vi "Stoerungen (449-512) - TRE08.vi"(8 "Fehler (Eingang)":errorcluster caption="Fehler (Eingang, kein Fehler)") -> (0 "Fehler (Ausgang)":errorcluster, 3 "Störungen 449-512":u64)   [LabVIEW 2015, in "Stoerungen.lvlib"]
uses:
  Stoerungen.lvlib
  PNS/Parameternamen PNS.ctl
  PNS/PNS.lvlib
  Stoerungen Messgeraet/Aktionen Kommunikation Stoerung.ctl
  Seiten/System Einstellungen/System Einstellungen.lvlib
  Seiten/System Einstellungen/Aktioen FGV System.ctl
  PNS/Aktionen FGV Istwerte.ctl
  cRIO/Stoermeldungen/Stoerungen 449-512.ctl
  cRIO/Stoermeldungen/Stoermeldungen.lvlib
panel:
  # "Störmeldungen PNS (449-512)"
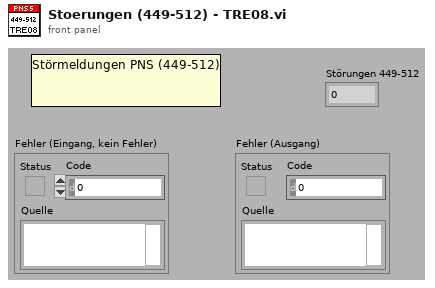
[diagram p1: front panel]
types:
  T1 = typedef "System Einstellungen.lvlib/Aktioen FGV System.ctl" = enum16{"lesen", "laden", "speichern", "Optionen schreiben", "Zeitstempel", "Reset BMP", "Reset SQP", "Wartung"}
  T2 = typedef "System Einstellungen.lvlib/Optionen.ctl" = cluster{"Störmeldep.":bool, "Betriebszustände":bool, "LN2 Befüllung":bool, "Klimaanlage ?":bool, "AK in ppm":bool, "log Cal-Gas":bool, "log 0-Gas":bool, "log CG zu PNS":bool, "Reserve":bool, "Reserve1":bool, "PNS?":bool, "Container":bool, "Mit N2 spülen":bool, "Span Gas Auswahl":T3, "VFS 1":bool, "VFS 2":bool, "VFS 3":bool, "VFS 4":bool, "TRE08":bool}
  T3 = typedef "Funktionstasten.lvlib/Spaneingang.ctl" = u16
  T4 = typedef "PNS.lvlib/Parameternamen PNS.ctl" = enum16{"Heizkreis 1", "Heizkreis 2", "Heizkreis 3", "Heizkreis 4", "Heizkreis 5", "Heizkreis 6", "Heizkreis 7", "Heizkreis 8"}
  T5 = typedef "PNS.lvlib/Aktionen FGV Istwerte.ctl" = enum16{"lesen", "initialisieren", "schreiben", "Störungen"}
  T6 = typedef "Stoerungen.lvlib/Aktionen Kommunikation Stoerung.ctl" = enum16{"lesen", "init", "FT-IR Komm", "FT-IR Betriebsart", "FT-IR Hintergrund", "cRIO Komm", "PNS Komm", "Dichtheitstest", "Life Bit", "FTIR Komm AK", "PMA Komm", "FID Komm", "PMA Cal", "FID Ch4 Cal", "FID THC Cal", "Cal Timeout", "VFS 1 Komm", "VFS 2 Komm", "VFS 3 Komm", "VFS 4 Komm", "TRE 08 Komm", "CG-Test vorzeitig", "CG-Test Span 1", "CG-Test Span 2", "CG-Test Span 3", "CG-Test Messgas", "CG-Test löschen", "Test", "Amium AK"}
  T7 = typedef "Stoermeldungen.lvlib/Stoerungen 449-512.ctl" = cluster{"ERR. 449":bool, "ERR. 450":bool, "ERR. 451":bool, "ERR. 452":bool, "ERR. 453":bool, "ERR. 454":bool, "ERR. 455":bool, "ERR. 456":bool, "ERR. 457":bool, "ERR. 458":bool, "ERR. 459":bool, "ERR. 460":bool, "ERR. 461":bool, "ERR. 462":bool, "ERR. 463":bool, "ERR. 464":bool, "ERR. 465":bool, "ERR. 466":bool, "ERR. 467":bool, "ERR. 468":bool, "ERR. 469":bool, "ERR. 470":bool, "ERR. 471":bool, "ERR. 472":bool, "ERR. 473":bool, "ERR. 474":bool, "ERR. 475":bool, "ERR. 476":bool, "ERR. 477":bool, "ERR. 478":bool, "ERR. 479":bool, "ERR. 480":bool, "ERR. 481":bool, "ERR. 482":bool, "ERR. 483":bool, "ERR. 484":bool, "ERR. 485":bool, "ERR. 486":bool, "ERR. 487":bool, "ERR. 488":bool, "ERR. 489":bool, "ERR. 490":bool, "ERR. 491":bool, "ERR. 492":bool, "ERR. 493":bool, "ERR. 494":bool, "ERR. 495":bool, "ERR. 496":bool, "ERR. 497":bool, "ERR. 498":bool, "ERR. 499":bool, "ERR. 500":bool, "ERR. 501":bool, "ERR. 502":bool, "ERR. 503":bool, "ERR. 504":bool, "ERR. 505":bool, "ERR. 506":bool, "ERR. 507":bool, "ERR. 508":bool, "ERR. 509":bool, "ERR. 510":bool, "ERR. 511":bool, "ERR. 512":bool}
  T8 = typedef "Steuerung PNS.lvclass/Regler.ctl" = cluster{"Istwert":i16, "Sollwert":i16, "Alarm MIN":i16, "Alarm MAX":i16, "Regler sperren":i16, "Analog Ausgang":i16}[]
  T9 = cluster{"Istwert":i16, "Sollwert":i16, "Alarm MIN":i16, "Alarm MAX":i16, "Regler sperren":i16, "Analog Ausgang":i16}
  T10 = typedef "Stoerungen.lvlib/Stoerungen Messgeraete.ctl" = cluster{"FT-IR Komm":bool, "FT-IR Betriebsart":bool, "FT-IR Hintergrundscan":bool, "Dichtheitstest":bool, "cRIO Komm":bool, "PNS Komm":bool, "Life Bit":bool, "FT-IR AK Komm":bool, "PMA Komm":bool, "FID Komm":bool, "PMA Cal":bool, "FID CH4 Cal":bool, "FID THC Cal":bool, "Cal Timeout":bool, "VFS 1 Komm":bool, "VFS 2 Komm":bool, "VFS 3 Komm":bool, "VFS 4 Komm":bool, "TRE 08 Komm":bool, "CG-Test":bool, "CG-Test 1":bool, "CG-Test 2":bool, "CG-Test 3":bool, "Messgas - Eingang":bool, "Amium AK Komm":bool}
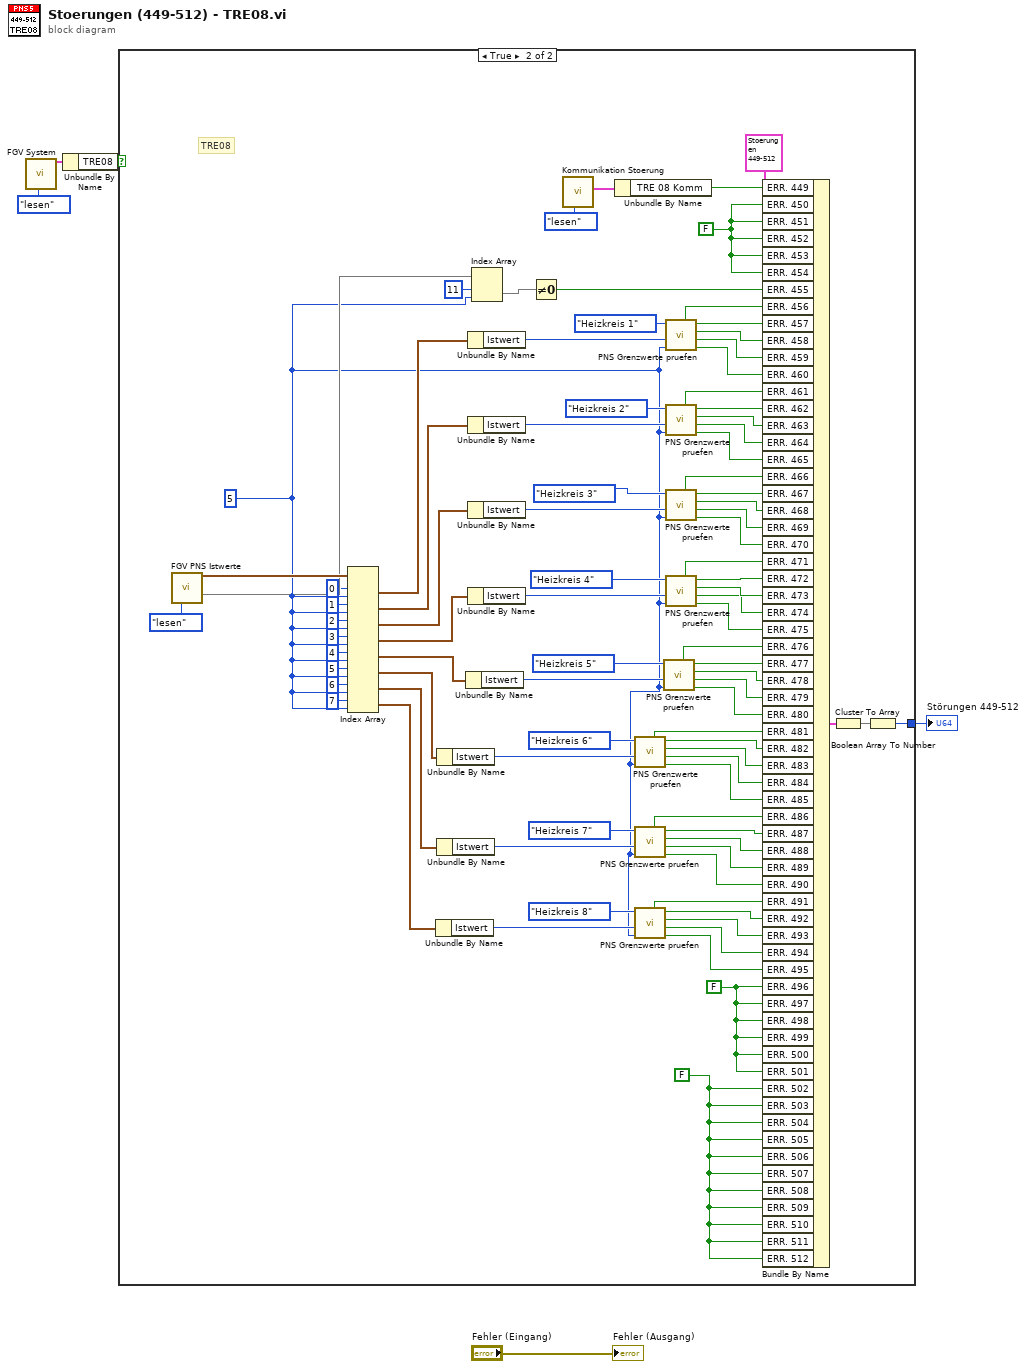
[diagram p0: block diagram]
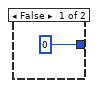
[diagram p2: hidden frame]
diagram:
  n1 = call "FGV System.vi"("Aktionen"=Aktioen_FGV_System."lesen") -> ("Optionen"=w3:T2)  [unwired: 13 in, 5 out]
  n2 = Unbundle By Name(w3) -> ("TRE08"=w1:bool)
  n3 = case shown="True" w1 {
    tunnel: [u64 0 w55] -> w4
    frame False {
    }
    frame True {
      w7 = 5 ("Deaktivierter Index (Spalte)")
      w54 = FALSE ("ERR. 240")
      w62 = FALSE ("ERR. 194")
      w60 = FALSE ("ERR. 194")
      # "TRE08"
      n4 = call "FGV PNS Istwerte.vi"("Aktionen"=Aktionen_FGV_Istwerte."lesen") -> ("Regler"=w92:T8, 10:w59)  [unwired: 10 in, 3 out]
      n5 = Index Array(array=w92, index (row) #1=0 ("Deaktivierter Index (Zeile)"), index (col) #1=w7, index (row) #2=1 ("Deaktivierter Index (Zeile)"), index (col) #2=w7, index (row) #3=2 ("Deaktivierter Index (Zeile)"), index (col) #3=w7, index (row) #4=3 ("Deaktivierter Index (Zeile)"), index (col) #4=w7, index (row) #5=4 ("Deaktivierter Index (Zeile)"), index (col) #5=w7, index (row) #6=5 ("Deaktivierter Index (Zeile)"), index (col) #6=w7, index (row) #7=6 ("Deaktivierter Index (Zeile)"), index (col) #7=w7, index (row) #8=7 ("Deaktivierter Index (Zeile)"), index (col) #8=w7) -> (element #1=w91:T9, element #2=w89:T9, element #3=w88:T9, element #4=w87:T9, element #5=w48:T9, element #6=w42:T9, element #7=w41:T9, element #8=w40:T9)
      n6 = Unbundle By Name(w40) -> ("Istwert"=w19:i16)
      n7 = Unbundle By Name(w42) -> ("Istwert"=w20:i16)
      n8 = Unbundle By Name(w41) -> ("Istwert"=w21:i16)
      n9 = Unbundle By Name(w48) -> ("Istwert"=w17:i16)
      n10 = Unbundle By Name(w91) -> ("Istwert"=w90:i16)
      n11 = Unbundle By Name(w89) -> ("Istwert"=w51:i16)
      n12 = Unbundle By Name(w88) -> ("Istwert"=w86:i16)
      n13 = Unbundle By Name(w87) -> ("Istwert"=w85:i16)
      n14 = Index Array(array=w59, index (row)=11 ("Index"), index (col)=w7) -> (element=w57)
      n15 = Not Equal To 0?(x=w57) -> (x != 0?=w56:bool)
      n16 = call "Kommunikation Stoerung.vi"("Aktionen"=Aktionen_Kommunikation_Stoerung."lesen") -> ("Störung Messgerät"=w64:T10)  [unwired: 10 in]
      n17 = Unbundle By Name(w64) -> ("TRE 08 Komm"=w61:bool)
      n18 = call "PNS Grenzwerte pruefen.vi"("Option"=w7, "Wert"=w20, "Parameternamen PNS"=Parameternamen_PNS."Heizkreis 6") -> ("AbschMax"=w35:bool, "AbschMin"=w36:bool, "WarnMax"=w37:bool, "WarnMin"=w38:bool, "F.Br."=w39:bool)  [unwired: 4 in]
      n19 = call "PNS Grenzwerte pruefen.vi"("Option"=w7, "Wert"=w21, "Parameternamen PNS"=Parameternamen_PNS."Heizkreis 7") -> ("AbschMax"=w30:bool, "AbschMin"=w31:bool, "WarnMax"=w32:bool, "WarnMin"=w33:bool, "F.Br."=w34:bool)  [unwired: 4 in]
      n20 = call "PNS Grenzwerte pruefen.vi"("Option"=w7, "Wert"=w19, "Parameternamen PNS"=Parameternamen_PNS."Heizkreis 8") -> ("AbschMax"=w25:bool, "AbschMin"=w26:bool, "WarnMax"=w27:bool, "WarnMin"=w28:bool, "F.Br."=w29:bool)  [unwired: 4 in]
      n21 = call "PNS Grenzwerte pruefen.vi"("Option"=w7, "Wert"=w17, "Parameternamen PNS"=Parameternamen_PNS."Heizkreis 5") -> ("AbschMax"=w43:bool, "AbschMin"=w44:bool, "WarnMax"=w45:bool, "WarnMin"=w46:bool, "F.Br."=w47:bool)  [unwired: 4 in]
      n22 = call "PNS Grenzwerte pruefen.vi"("Option"=w7, "Wert"=w90, "Parameternamen PNS"=Parameternamen_PNS."Heizkreis 1") -> ("AbschMax"=w80:bool, "AbschMin"=w81:bool, "WarnMax"=w82:bool, "WarnMin"=w83:bool, "F.Br."=w84:bool)  [unwired: 4 in]
      n23 = call "PNS Grenzwerte pruefen.vi"("Option"=w7, "Wert"=w51, "Parameternamen PNS"=Parameternamen_PNS."Heizkreis 2") -> ("AbschMax"=w75:bool, "AbschMin"=w76:bool, "WarnMax"=w77:bool, "WarnMin"=w78:bool, "F.Br."=w79:bool)  [unwired: 4 in]
      n24 = call "PNS Grenzwerte pruefen.vi"("Option"=w7, "Wert"=w86, "Parameternamen PNS"=Parameternamen_PNS."Heizkreis 3") -> ("AbschMax"=w70:bool, "AbschMin"=w71:bool, "WarnMax"=w72:bool, "WarnMin"=w73:bool, "F.Br."=w74:bool)  [unwired: 4 in]
      n25 = call "PNS Grenzwerte pruefen.vi"("Option"=w7, "Wert"=w85, "Parameternamen PNS"=Parameternamen_PNS."Heizkreis 4") -> ("AbschMax"=w65:bool, "AbschMin"=w66:bool, "WarnMax"=w67:bool, "WarnMin"=w68:bool, "F.Br."=w69:bool)  [unwired: 4 in]
      n26 = Bundle By Name(cluster=T7 {"ERR. 449"=FALSE, "ERR. 450"=FALSE, "ERR. 451"=FALSE, "ERR. 452"=FALSE, "ERR. 453"=FALSE, "ERR. 454"=FALSE, "ERR. 455"=FALSE, "ERR. 456"=FALSE, "ERR. 457"=FALSE, "ERR. 458"=FALSE, "ERR. 459"=FALSE, "ERR. 460"=FALSE, "ERR. 461"=FALSE, "ERR. 462"=FALSE, "ERR. 463"=FALSE, "ERR. 464"=FALSE, "ERR. 465"=FALSE, "ERR. 466"=FALSE, "ERR. 467"=FALSE, "ERR. 468"=FALSE, "ERR. 469"=FALSE, "ERR. 470"=FALSE, "ERR. 471"=FALSE, "ERR. 472"=FALSE, "ERR. 473"=FALSE, "ERR. 474"=FALSE, "ERR. 475"=FALSE, "ERR. 476"=FALSE, "ERR. 477"=FALSE, "ERR. 478"=FALSE, "ERR. 479"=FALSE, "ERR. 480"=FALSE, "ERR. 481"=FALSE, "ERR. 482"=FALSE, "ERR. 483"=FALSE, "ERR. 484"=FALSE, "ERR. 485"=FALSE, "ERR. 486"=FALSE, "ERR. 487"=FALSE, "ERR. 488"=FALSE, "ERR. 489"=FALSE, "ERR. 490"=FALSE, "ERR. 491"=FALSE, "ERR. 492"=FALSE, "ERR. 493"=FALSE, "ERR. 494"=FALSE, "ERR. 495"=FALSE, "ERR. 496"=FALSE, "ERR. 497"=FALSE, "ERR. 498"=FALSE, "ERR. 499"=FALSE, "ERR. 500"=FALSE, "ERR. 501"=FALSE, "ERR. 502"=FALSE, "ERR. 503"=FALSE, "ERR. 504"=FALSE, "ERR. 505"=FALSE, "ERR. 506"=FALSE, "ERR. 507"=FALSE, "ERR. 508"=FALSE, "ERR. 509"=FALSE, "ERR. 510"=FALSE, "ERR. 511"=FALSE, "ERR. 512"=FALSE} ("STÖRUNGEN 193-256"), "ERR. 449"=w61, "ERR. 450"=w60, "ERR. 451"=w60, "ERR. 452"=w60, "ERR. 453"=w60, "ERR. 454"=w60, "ERR. 455"=w56, "ERR. 456"=w84, "ERR. 457"=w83, "ERR. 458"=w82, "ERR. 459"=w81, "ERR. 460"=w80, "ERR. 461"=w79, "ERR. 462"=w78, "ERR. 463"=w77, "ERR. 464"=w76, "ERR. 465"=w75, "ERR. 466"=w74, "ERR. 467"=w73, "ERR. 468"=w72, "ERR. 469"=w71, "ERR. 470"=w70, "ERR. 471"=w69, "ERR. 472"=w68, "ERR. 473"=w67, "ERR. 474"=w66, "ERR. 475"=w65, "ERR. 476"=w47, "ERR. 477"=w46, "ERR. 478"=w45, "ERR. 479"=w44, "ERR. 480"=w43, "ERR. 481"=w39, "ERR. 482"=w38, "ERR. 483"=w37, "ERR. 484"=w36, "ERR. 485"=w35, "ERR. 486"=w34, "ERR. 487"=w33, "ERR. 488"=w32, "ERR. 489"=w31, "ERR. 490"=w30, "ERR. 491"=w29, "ERR. 492"=w28, "ERR. 493"=w27, "ERR. 494"=w26, "ERR. 495"=w25, "ERR. 496"=w54, "ERR. 497"=w54, "ERR. 498"=w54, "ERR. 499"=w54, "ERR. 500"=w54, "ERR. 501"=w54, "ERR. 502"=w62, "ERR. 503"=w62, "ERR. 504"=w62, "ERR. 505"=w62, "ERR. 506"=w62, "ERR. 507"=w62, "ERR. 508"=w62, "ERR. 509"=w62, "ERR. 510"=w62, "ERR. 511"=w62, "ERR. 512"=w62) -> (w95:T7)
      n27 = Cluster To Array(cluster=w95) -> (array=w94:bool[])
      n28 = Boolean Array To Number ("Boolesches Array nach Zahl")(Boolean array=w94) -> (number=w55:u64)
    }
  }
  "Störungen 449-512" <- w4
  "Fehler (Ausgang)" <- "Fehler (Eingang)"
